vi "Lidar PT.vi"() -> (0 "error out":errorcluster={"status"=FALSE, "code"=0, "source"="i2clib_write.vi<ERR>\nDevice or resource busy\n\n\n<b>Complete call chain:</b>\n     i2clib_write.vi\n     WPI_I2CWrite.vi\n     Periodic Tasks.vi\n     Robot Main.vi"}, 2 "x != 0?":bool, 3 "*(type *) &x":i16)   [LabVIEW 2014]
uses:
  <vilib>/Rock Robotics/SystemInterfaces/i2clib/i2c_bus.ctl
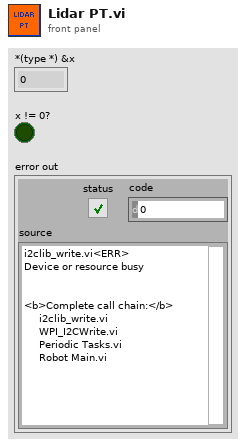
[diagram p1: front panel]
types:
  T1 = typedef "i2c_bus.ctl" = enum16{"I2C On-Board", "I2C MXP", "Invalid"}
  T2 = typedef "WPI_I2CDevRef.ctl" = cluster{"DevStatus":errorcluster, "Controller":T3, "Device Address":u8, "Handle":i32, "I2C Bus":T1}
  T3 = typedef "FPGA_TypedefDigitalModule.ctl" = enum16{"Controller 1"}
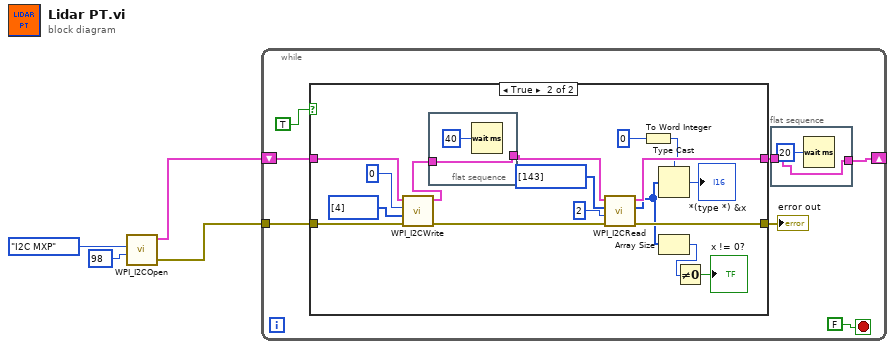
[diagram p0: block diagram]
diagram:
  n1 = call <vilib>:"WPI_I2COpen.vi"("Device Address"=u8 98, "I2C Bus"=i2c_bus."I2C MXP") -> ("error out"=w3:errorcluster, "I2CDevRef"=w4:T2)  [unwired: 8 in]
  n2 = while {
    shift-right: [w6] -> _
    shift-left: w4 -> [w9]
    tunnel: w3 -> [w8]
    stop <- FALSE stop-if-true
    n3 = case shown="True" TRUE ("Send") {
      tunnel: w9 -> [w15 w29]
      tunnel: [w15 w26] -> w5
      tunnel: w8 -> [w14 w28]
      tunnel: [w14 w27] -> w7
      frame False {
      }
      frame True {
        n4 = call <vilib>:"WPI_I2CWrite.vi"("error in (no error)"=w28, "I2CDataToSend"=u8[] [4], "I2CRegister"=u8 0, "I2CDevRef"=w29) -> ("error out"=w32:errorcluster, "I2CDevRef"=w22:T2)  [unwired: 6 in]
        n5 = flat-sequence {
          tunnel: w22 -> [w33]
          tunnel: [w33] -> w21
          frame #0 {
            n6 = Wait (ms)(milliseconds to wait=u32 40) -> ()  [unwired: 1 out]
          }
        }
        n7 = call <vilib>:"WPI_I2CRead.vi"("error in (no error)"=w32, "I2CBytesToRead"=u8 2 ("Read Size"), "I2CRegister"=u8[] [143], "I2CDevRef"=w21) -> ("error out"=w27:errorcluster, "Data Out"=w19:u8[], "I2CDevRef"=w26:T2)  [unwired: 5 in]
        n8 = To Word Integer(number=i16 0) -> (16bit integer=w18:i16)
        n9 = Type Cast(type=w18, x=w19) -> (*(type *) &x=→"*(type *) &x":i16)
        n10 = Array Size(array=w19) -> (size(s)=w23:i32)
        n11 = Not Equal To 0?(x=w23) -> (x != 0?=→"x != 0?":bool)
      }
    }
    "error out" <- w7
    n12 = flat-sequence {
      tunnel: [w12] -> w6
      tunnel: w5 -> [w12]
      frame #0 {
        n13 = Wait (ms)(milliseconds to wait=u32 20) -> ()  [unwired: 1 out]
      }
    }
  }
